vi "Parameters 2 Step ID.vi"(0 "Setpoint 3":dbl format="%#_13g", 1 "ID List":string[](array[string]), 5 "Parameter 1":i32, 7 "Setpoint 1":dbl format="%#_13g", 9 "Parameter 2":i32, 11 "Setpoint 2":dbl format="%#_13g", 12 "Parameter 3":i32, 13 "StepIndex":i32) -> (8 "Step ID":string)   [LabVIEW 2013]
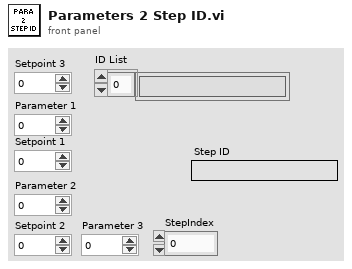
[diagram p1: front panel]
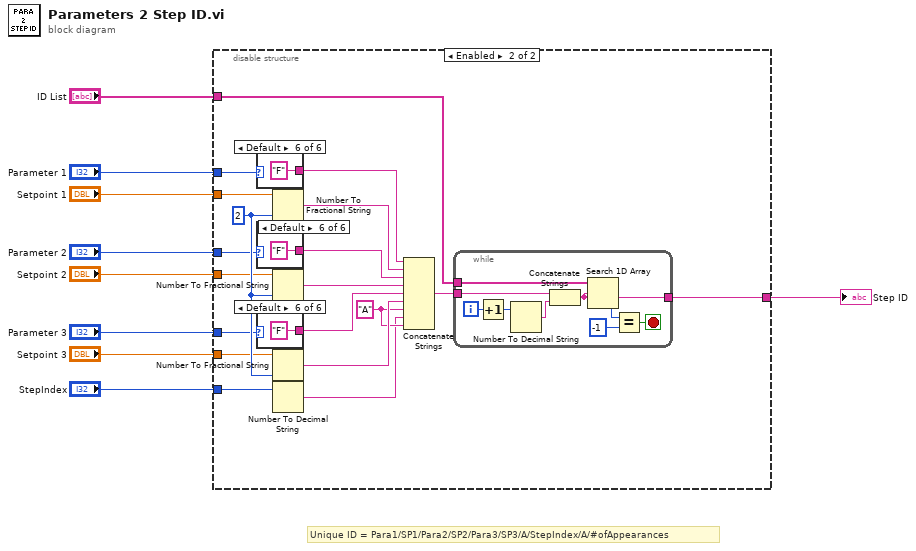
[diagram p0: block diagram]
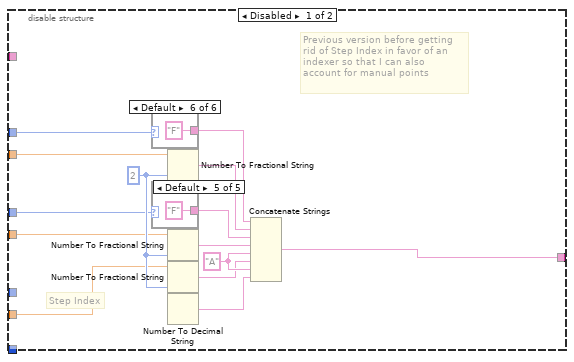
[diagram p2: hidden frame]
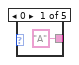
[diagram p3: hidden frame]
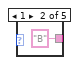
[diagram p4: hidden frame]
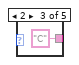
[diagram p5: hidden frame]
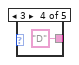
[diagram p6: hidden frame]
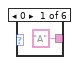
[diagram p7: hidden frame]
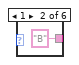
[diagram p8: hidden frame]
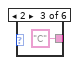
[diagram p9: hidden frame]
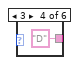
[diagram p10: hidden frame]
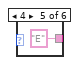
[diagram p11: hidden frame]
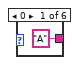
[diagram p12: hidden frame]
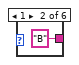
[diagram p13: hidden frame]
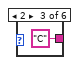
[diagram p14: hidden frame]
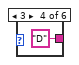
[diagram p15: hidden frame]
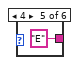
[diagram p16: hidden frame]
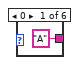
[diagram p17: hidden frame]
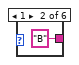
[diagram p18: hidden frame]
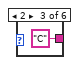
[diagram p19: hidden frame]
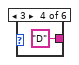
[diagram p20: hidden frame]
diagram:
  # "Unique ID = Para1/SP1/Para2/SP2/Para3/SP3/A/StepIndex/A/#ofAppearances"
  n1 = disable-structure shown="Enabled" {
    disable-tunnel: "Parameter 1" -> [w16 w49]
    disable-tunnel: "Setpoint 1" -> [w15 w48]
    disable-tunnel: "Parameter 2" -> [w14 w39]
    disable-tunnel: "Setpoint 2" -> [w13 w47]
    disable-tunnel: "Setpoint 3" -> [w12 w46]
    disable-tunnel: [w10 w43] -> w4
    disable-tunnel: "ID List" -> [_ w45]
    disable-tunnel: "StepIndex" -> [_ w42]
    disable-tunnel: "Parameter 3" -> [_ w37]
    frame Disabled {
      w24 = "A" ("string")
      w21 = i16 2 ("width (-)")
      # "Step Index"
      # "Previous version before getting\nrid of Step Index in favor of an\nindexer so that I can also\naccount for manual points"
      n2 = case shown="Default" w16 {
        tunnel: ["A" "B" "C" "D" "E" "F"] -> w20
        frame 0 {
        }
        frame 1 {
        }
        frame 2 {
        }
        frame 3 {
        }
        frame 4 {
        }
        frame Default {
        }
      }
      n3 = case shown="Default" w14 {
        tunnel: ["A" "B" "C" "D" "F"] -> w18
        frame 0 {
        }
        frame 1 {
        }
        frame 2 {
        }
        frame 3 {
        }
        frame Default {
        }
      }
      n4 = Number To Fractional String(number=w15, precision (6)=w21) -> (F-format string=w19:string)  [unwired: 2 in]
      n5 = Number To Fractional String(number=w13, precision (6)=w21) -> (F-format string=w17:string)  [unwired: 2 in]
      n6 = Number To Fractional String(number=w12, precision (6)=w21) -> (F-format string=w23:string)  [unwired: 2 in]
      n7 = Number To Decimal String() -> (number=w11:i32, decimal integer string=w22:string)  [unwired: 1 in]
      n8 = Concatenate Strings(w20, w19, w18, w17, w24, w23, w24, w22) -> (w10:string)
    }
    frame Enabled {
      w41 = "A" ("string")
      w53 = i16 2 ("width (-)")
      n9 = case shown="Default" w49 {
        tunnel: ["A" "B" "C" "D" "E" "F"] -> w52
        frame 0 {
        }
        frame 1 {
        }
        frame 2 {
        }
        frame 3 {
        }
        frame 4 {
        }
        frame Default {
        }
      }
      n10 = case shown="Default" w39 {
        tunnel: ["A" "B" "C" "D" "E" "F"] -> w38
        frame 0 {
        }
        frame 1 {
        }
        frame 2 {
        }
        frame 3 {
        }
        frame 4 {
        }
        frame Default {
        }
      }
      n11 = case shown="Default" w37 {
        tunnel: ["A" "B" "C" "D" "E" "F"] -> w36
        frame 0 {
        }
        frame 1 {
        }
        frame 2 {
        }
        frame 3 {
        }
        frame 4 {
        }
        frame Default {
        }
      }
      n12 = Number To Fractional String(number=w48, precision (6)=w53) -> (F-format string=w51:string)  [unwired: 2 in]
      n13 = Number To Fractional String(number=w47, precision (6)=w53) -> (F-format string=w50:string)  [unwired: 2 in]
      n14 = Number To Fractional String(number=w46, precision (6)=w53) -> (F-format string=w54:string)  [unwired: 2 in]
      n15 = Number To Decimal String(number=w42) -> (decimal integer string=w40:string)  [unwired: 1 in]
      n16 = Concatenate Strings(w52, w51, w38, w50, w36, w54, w41, w40, w41) -> (w44:string)
      n17 = while {
        tunnel: w45 -> [w75]
        tunnel: w44 -> [w72]
        tunnel: [w70] -> w43
        i -> [w74]
        stop <- w67 stop-if-true
        n18 = Increment(x=w74) -> (x+1=w73:i32)
        n19 = Number To Decimal String(number=w73) -> (decimal integer string=w71:string)  [unwired: 1 in]
        n20 = Concatenate Strings(w72, w71) -> (w70:string)
        n21 = Search 1D Array(1D array=w75, element=w70) -> (index of element=w69:i32)  [unwired: 1 in]
        n22 = Equal?(x=w69, y=-1) -> (x = y?=w67:bool)
      }
    }
  }
  "Step ID" <- w4
